vi "write_channel_commands.vi"(8 "Input 2 Settings":T1 {"Threshold (V)" min=-2.5 max=2.5 step=0.001}, 9 "Input 1 Settings":T1 {"Threshold (V)" min=-2.5 max=2.5 step=0.001}, 10 "Trig Channel Settings":T1 {"Threshold (V)" min=-2.5 max=2.5 step=0.001}, 11 "Gate Channel Settings":T1 {"Threshold (V)" min=-2.5 max=2.5 step=0.001}) -> (2 "Command Out":string)   [LabVIEW 2015]
uses:
  Controls/MCS/mcs_channel.ctl
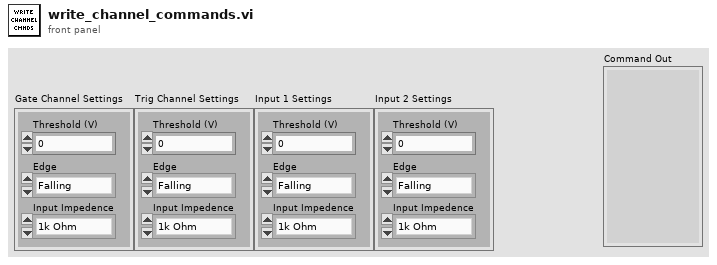
[diagram p1: front panel]
types:
  T1 = typedef "mcs_channel.ctl" = cluster{"Threshold (V)":dbl, "Edge":enum16{"Falling", "Rising"}, "Input Impedence":enum16{"1k Ohm", "50 Ohm"}}
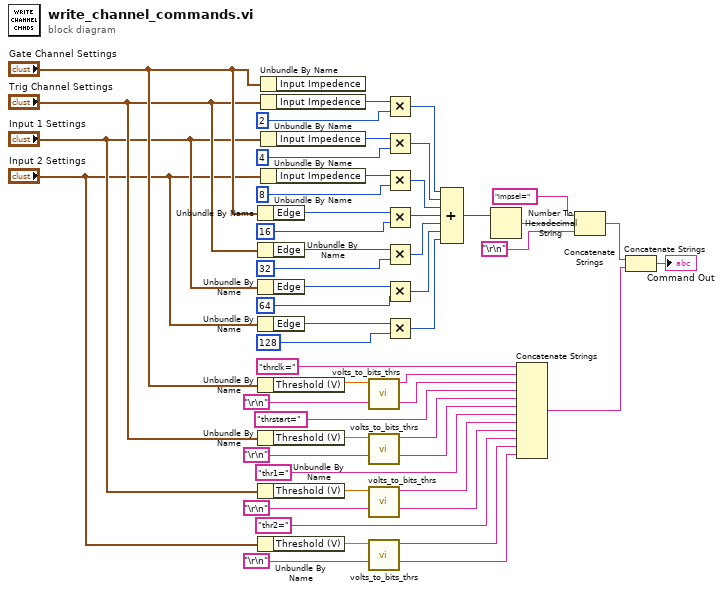
[diagram p0: block diagram]
diagram:
  n1 = Unbundle By Name("Gate Channel Settings") -> ("Edge"=w42:enum16{"Falling", "Rising"})
  n2 = Unbundle By Name("Trig Channel Settings") -> ("Edge"=w40:enum16{"Falling", "Rising"})
  n3 = Unbundle By Name("Input 1 Settings") -> ("Edge"=w38:enum16{"Falling", "Rising"})
  n4 = Unbundle By Name("Input 2 Settings") -> ("Edge"=w36:enum16{"Falling", "Rising"})
  n5 = Unbundle By Name("Gate Channel Settings") -> ("Threshold (V)"=w19:dbl)
  n6 = Unbundle By Name("Trig Channel Settings") -> ("Threshold (V)"=w18:dbl)
  n7 = Unbundle By Name("Input 1 Settings") -> ("Threshold (V)"=w17:dbl)
  n8 = Unbundle By Name("Input 2 Settings") -> ("Threshold (V)"=w16:dbl)
  n9 = Unbundle By Name("Gate Channel Settings") -> ()  [unwired: 1 out]
  n10 = Unbundle By Name("Trig Channel Settings") -> ("Input Impedence"=w48:enum16{"1k Ohm", "50 Ohm"})
  n11 = Unbundle By Name("Input 1 Settings") -> ("Input Impedence"=w47:enum16{"1k Ohm", "50 Ohm"})
  n12 = Unbundle By Name("Input 2 Settings") -> ("Input Impedence"=w46:enum16{"1k Ohm", "50 Ohm"})
  n13 = call "volts_to_bits_thrs.vi"("Voltage"=w19) -> ("Bits"=w14:string)  [unwired: 10 in]
  n14 = call "volts_to_bits_thrs.vi"("Voltage"=w18) -> ("Bits"=w11:string)  [unwired: 10 in]
  n15 = call "volts_to_bits_thrs.vi"("Voltage"=w17) -> ("Bits"=w8:string)  [unwired: 10 in]
  n16 = call "volts_to_bits_thrs.vi"("Voltage"=w16) -> ("Bits"=w5:string)  [unwired: 10 in]
  n17 = Multiply(x=w48, y=2) -> (x*y=w34:i32)
  n18 = Multiply(x=w47, y=4) -> (x*y=w33:i32)
  n19 = Multiply(x=w46, y=8) -> (x*y=w32:i32)
  n20 = Multiply(x=w42, y=16) -> (x*y=w31:i32)
  n21 = Multiply(x=w40, y=32) -> (x*y=w30:i32)
  n22 = Multiply(x=w38, y=64) -> (x*y=w29:i32)
  n23 = Multiply(x=w36, y=128) -> (x*y=w28:i32)
  n24 = Compound Arithmetic op=ADD(w34, w33, w32, w31, w30, w29, w28) -> (w27:i32)
  n25 = Number To Hexadecimal String(2:w27) -> (0:w25:string)  [unwired: 1 in]
  n26 = Concatenate Strings("thrclk=", w14, "\r\n", "thrstart=", w11, "\r\n", "thr1=", w8, "\r\n", "thr2=", w5, "\r\n") -> (w2:string)
  n27 = Concatenate Strings("impsel=" ("string"), w25, "\r\n") -> (w3:string)
  n28 = Concatenate Strings(w3, w2) -> (→"Command Out":string)
